vi "Update Class Info.vi"(8 "error in (no error)":errorcluster, 10 "Item ID":string, 11 "Customer DAO JSON in":refnum<class "Object DAO JSON.lvclass">) -> (0 "error out":errorcluster, 2 "Item Updated?":bool, 3 "Customer DAO JSON out":refnum<class "Object DAO JSON.lvclass">)   [LabVIEW 2020, in "Object DAO JSON.lvclass"]
uses:
  Object DAO JSON.lvclass
  C:/Users/fflores/Desktop/DataBase - Copy - Copy - Copy/Object DAO/Object DAO.lvclass
  Object DAO JSON.lvclass/Object DAO JSON.ctl
  Object DAO/Object DAO.lvclass/Object DAO.ctl
  Object DAO/Member Accessors/Get Object Information.vi
  <vilib>/JDP Science/JSONtext/JSONtext.lvlib
  External Libraries/JSON File Manipulation.lvlibp
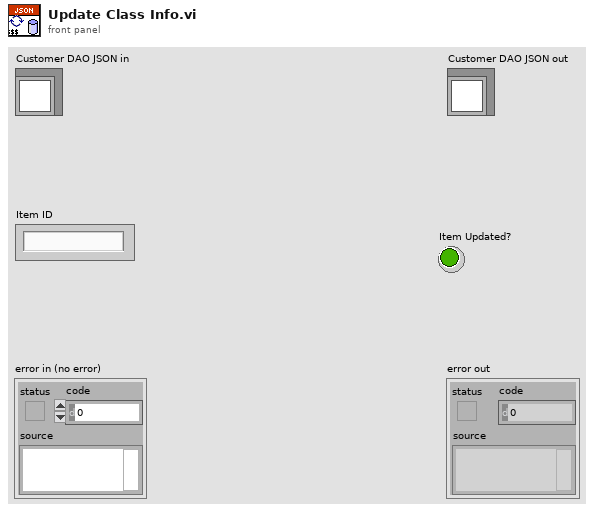
[diagram p1: front panel]
types:
  T1 = typedef "Object DAO.lvclass/Object Information.ctl" = cluster{"String":string, "Boolean":bool, "Numeric":dbl, "id":string}
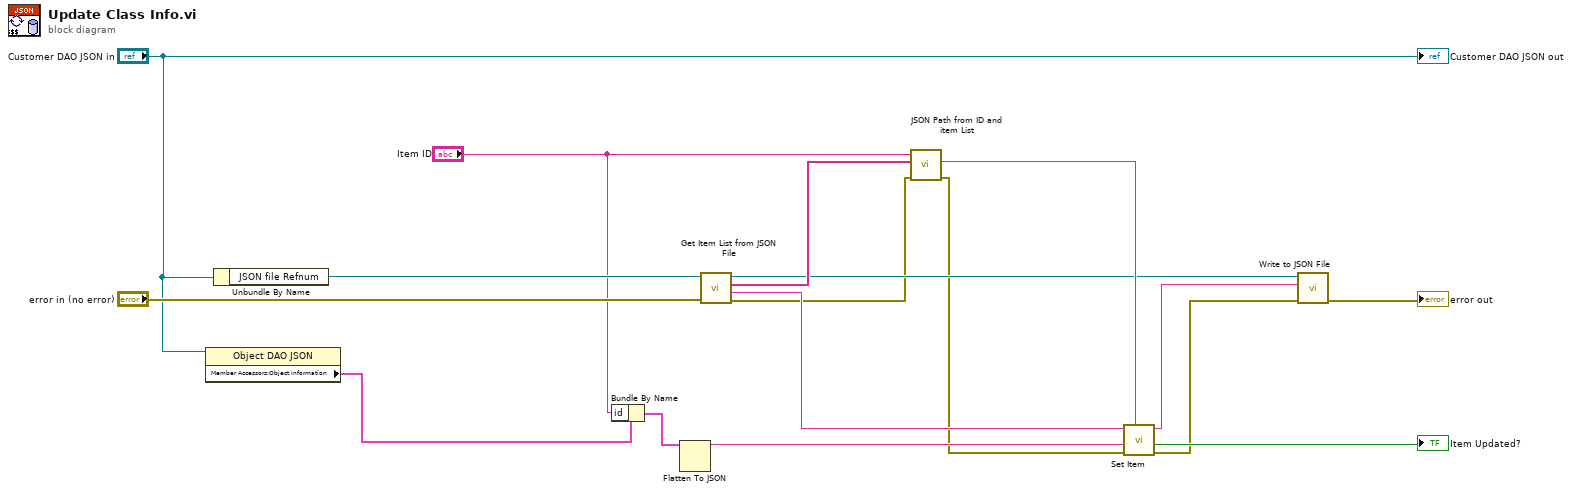
[diagram p0: block diagram]
diagram:
  n1 = property class="Object DAO JSON"(reference="Customer DAO JSON in") -> ("Member Accessors:Object Information"=w1:T1)  [unwired: 1 in, 2 out]
  n2 = Unbundle By Name("Customer DAO JSON in") -> ("JSON file Refnum"=w11:refnum<file>)
  n3 = Bundle By Name(cluster=w1, "id"="Item ID") -> (w4:T1)
  n4 = Flatten To JSON(anything=w4) -> (JSON string=w13:string)  [unwired: 2 in, 1 out]
  n5 = call "Get Item List from JSON File.vi"("error in (no error)"="error in (no error)", "Byte Stream File in"=w11) -> ("error out"=w5:errorcluster, "JSON String"=w12:string, "Item List"=w17:string[], "Byte Stream File out"=w15:refnum<file>)  [unwired: 6 in]
  n6 = call "JSON Path from ID and item List.vi"("error in (no error)"=w5, "Item List"=w17, "Item ID"="Item ID") -> ("error out"=w7:errorcluster, "Item JSON string"=w16:string)  [unwired: 7 in]
  n7 = call <vilib>:"Set Item.vi"("$Path or Item Name"=w16, "error in (no error)"=w7, "JSON to Insert"=w13, "JSON"=w12) -> ("error out"=w6:errorcluster, "Replaced"=→"Item Updated?":bool, "<JSON>"=w14:string)  [unwired: 4 in]
  n8 = call "Write to JSON File.vi"("error in (no error)"=w6, "JSON String"=w14, "Byte Stream File in"=w15) -> ("error out"=→"error out":errorcluster)  [unwired: 8 in]
  "Customer DAO JSON out" <- "Customer DAO JSON in"
